vi "New Main Log Loop.vi"() -> ()   [LabVIEW 2015]
uses:
  packet types.ctl
  Main/Robot Global Data.vi
  <vilib>/Rock Robotics/WPI/Solenoid/Deprecated/WPI_SolenoidGetBool.vi
  <vilib>/Rock Robotics/WPI/Ultrasonic/WPI_SonarSRF04DigitalGetRange.vi
  <vilib>/Rock Robotics/WPI/Ultrasonic/WPI_UltrasonicRangeUnits.ctl
  <vilib>/Rock Robotics/WPI/CAN/Jaguar/SubVIs/WPI_CANJaguar_ControlMode.ctl
  <vilib>/Rock Robotics/WPI/CAN/TalonSRX/WPI_CANTalonSRX_APIControlMode.ctl
  <vilib>/Rock Robotics/SystemInterfaces/DIO/FPGA_DIOPWMChannel.ctl
  <vilib>/Rock Robotics/WPI/PWM/WPI_PWMDeadband.ctl
  <vilib>/Rock Robotics/WPI/MotorControl/WPI_MotorControlType.ctl
  <vilib>/Rock Robotics/WPI/MotorControl/WPI_MotorControlDeviceRef.ctl
  <vilib>/Rock Robotics/WPI/Solenoid/WPI_SolenoidChannel.ctl
  <vilib>/Rock Robotics/WPI/Solenoid/WPI_SolenoidDevRef.ctl
  <vilib>/Rock Robotics/SystemInterfaces/DIO/FPGA_DIOChannel.ctl
  <vilib>/Rock Robotics/SystemInterfaces/Counter/FPGA_CounterCtrSystemIndex.ctl
  <vilib>/Rock Robotics/WPI/Ultrasonic/WPI_UltrasonicDeviceRef.ctl
  <vilib>/Rock Robotics/WPI/Compressor/WPI_CompressorDevRef.ctl
panel:
  in  "UltrasonicDevRef 2":T1={"DevStatus"={"status"=FALSE, "code"=0, "source"=""}, "Ping Channel"=enum."Invalid", "Echo Channel"=enum."Invalid", "CntIndex"=enum."Invalid"}
  in  "CompressorDevRef":T4
  in  "UltrasonicDevRef":T1={"DevStatus"={"status"=FALSE, "code"=0, "source"=""}, "Ping Channel"=enum."Invalid", "Echo Channel"=enum."Invalid", "CntIndex"=enum."Invalid"}
  out "error out":errorcluster
  out "result string":string
  in  "Piston 2 & 3 Val":T5={"DevStatus"={"status"=FALSE, "code"=0, "source"=""}, "Pneumatics Control Module"=0, "Forward Solenoid Channel"=enum."Invalid", "Reverse Solenoid Channel"=enum."Invalid"}
  in  "Piston 1 Val":T5={"DevStatus"={"status"=FALSE, "code"=0, "source"=""}, "Pneumatics Control Module"=0, "Forward Solenoid Channel"=enum."Invalid", "Reverse Solenoid Channel"=enum."Invalid"}
  in  "Collector Motor":T7={"DeviceStatus"={"status"=FALSE, "code"=0, "source"=""}, "Type"=enum."PWM", "PWM"={"PWM Channel"=enum."Invalid", "DeadBand"={"Name"="", "maxPositivePwm"=0, "minPositivePwm"=0, "centerPwm"=0, "maxNegativePwm"=0, "minNegativePwm"=0, "angularRange"=0}}, "CAN"={"Device Number"=0, "Control Mode"=enum."Percent VBus", "Semaphore"=refnum, "Max Vout"=12.0, "TalonSRX Control Mode"=enum."Percent VBus"}, "Invert"=FALSE}
  in  "Left Drive Motor":T7={"DeviceStatus"={"status"=FALSE, "code"=0, "source"=""}, "Type"=enum."PWM", "PWM"={"PWM Channel"=enum."Invalid", "DeadBand"={"Name"="", "maxPositivePwm"=0, "minPositivePwm"=0, "centerPwm"=0, "maxNegativePwm"=0, "minNegativePwm"=0, "angularRange"=0}}, "CAN"={"Device Number"=0, "Control Mode"=enum."Percent VBus", "Semaphore"=refnum, "Max Vout"=12.0, "TalonSRX Control Mode"=enum."Percent VBus"}, "Invert"=FALSE}
  in  "Right Drive Motor":T7={"DeviceStatus"={"status"=FALSE, "code"=0, "source"=""}, "Type"=enum."PWM", "PWM"={"PWM Channel"=enum."Invalid", "DeadBand"={"Name"="", "maxPositivePwm"=0, "minPositivePwm"=0, "centerPwm"=0, "maxNegativePwm"=0, "minNegativePwm"=0, "angularRange"=0}}, "CAN"={"Device Number"=0, "Control Mode"=enum."Percent VBus", "Semaphore"=refnum, "Max Vout"=12.0, "TalonSRX Control Mode"=enum."Percent VBus"}, "Invert"=FALSE}
  in  "Right CAN Drive Motor":T7={"DeviceStatus"={"status"=FALSE, "code"=0, "source"=""}, "Type"=enum."PWM", "PWM"={"PWM Channel"=enum."PWM 1", "DeadBand"={"Name"="", "maxPositivePwm"=0, "minPositivePwm"=0, "centerPwm"=0, "maxNegativePwm"=0, "minNegativePwm"=0, "angularRange"=0}}, "CAN"={"Device Number"=0, "Control Mode"=enum."Percent VBus", "Semaphore"=refnum, "Max Vout"=12.0, "TalonSRX Control Mode"=enum."Percent VBus"}, "Invert"=FALSE}
  in  "Collector CAN Motor":T7={"DeviceStatus"={"status"=FALSE, "code"=0, "source"=""}, "Type"=enum."PWM", "PWM"={"PWM Channel"=enum."PWM 1", "DeadBand"={"Name"="", "maxPositivePwm"=0, "minPositivePwm"=0, "centerPwm"=0, "maxNegativePwm"=0, "minNegativePwm"=0, "angularRange"=0}}, "CAN"={"Device Number"=0, "Control Mode"=enum."Percent VBus", "Semaphore"=refnum, "Max Vout"=12.0, "TalonSRX Control Mode"=enum."Percent VBus"}, "Invert"=FALSE}
  in  "Left CAN Drive Motor":T7={"DeviceStatus"={"status"=FALSE, "code"=0, "source"=""}, "Type"=enum."PWM", "PWM"={"PWM Channel"=enum."PWM 1", "DeadBand"={"Name"="", "maxPositivePwm"=0, "minPositivePwm"=0, "centerPwm"=0, "maxNegativePwm"=0, "minNegativePwm"=0, "angularRange"=0}}, "CAN"={"Device Number"=0, "Control Mode"=enum."Percent VBus", "Semaphore"=refnum, "Max Vout"=12.0, "TalonSRX Control Mode"=enum."Percent VBus"}, "Invert"=FALSE}
  in  "error in (no error)":errorcluster
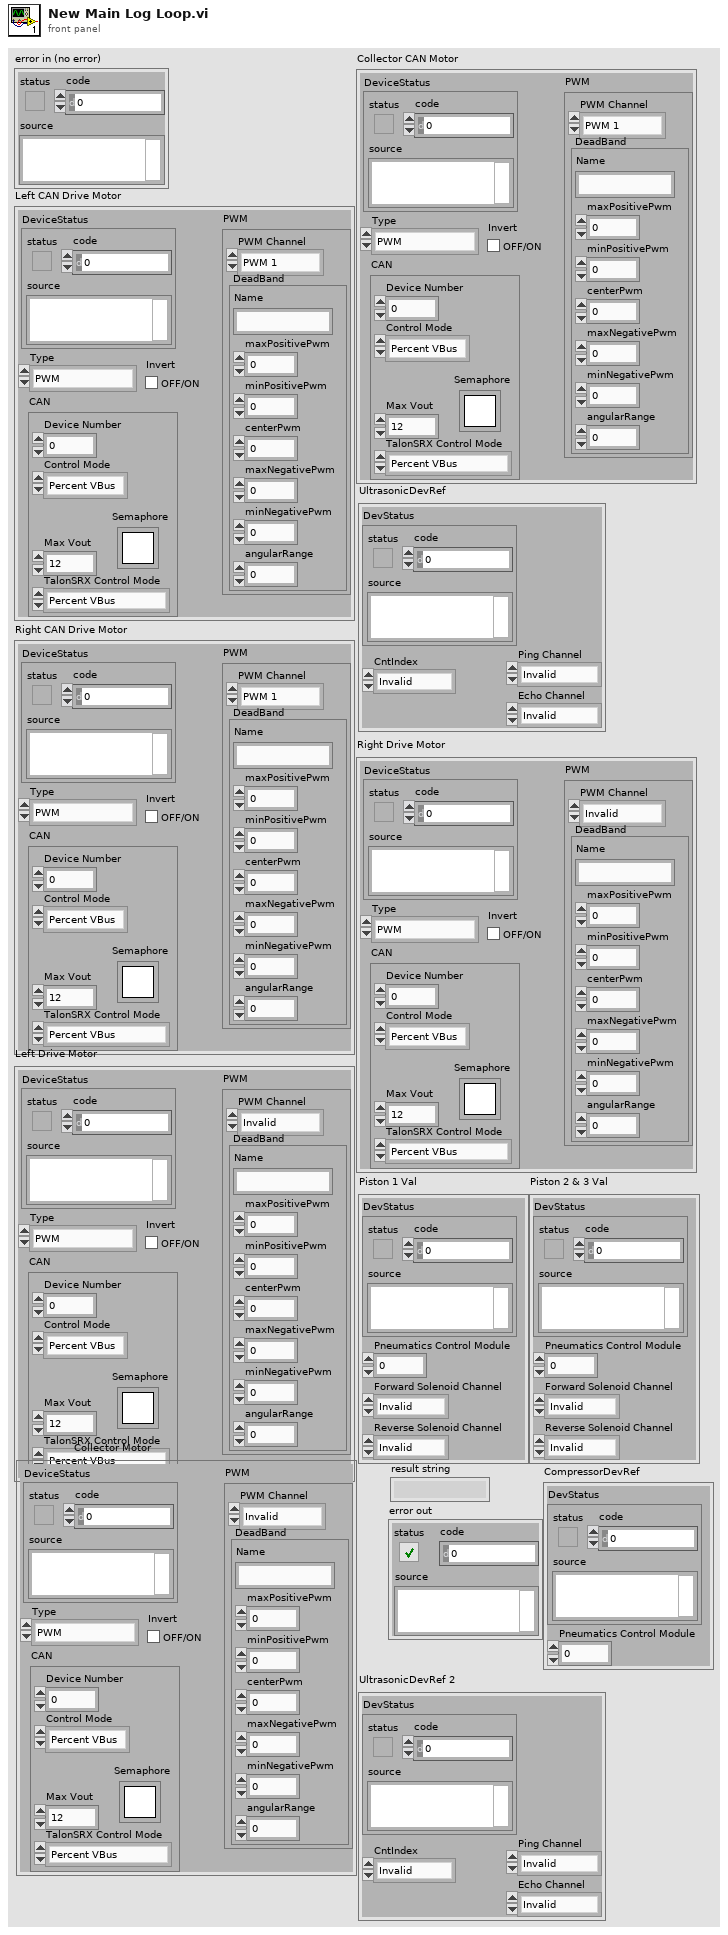
[diagram p1: front panel]
types:
  T1 = typedef "WPI_UltrasonicDeviceRef.ctl" = cluster{"DevStatus":errorcluster, "Ping Channel":T2, "Echo Channel":T2, "CntIndex":T3}
  T2 = typedef "FPGA_DIOChannel.ctl" = enum8{"DIO 0", "DIO 1", "DIO 2", "DIO 3", "DIO 4", "DIO 5", "DIO 6", "DIO 7", "DIO 8", "DIO 9", "DIO MXP 0", "DIO MXP 1", "DIO MXP 2", "DIO MXP 3", "DIO MXP 4", "DIO MXP 5", "DIO MXP 6", "DIO MXP 7", "DIO MXP 8", "DIO MXP 9", "DIO MXP 10", "DIO MXP 11", "DIO MXP 12", "DIO MXP 13", "DIO MXP 14", "DIO MXP 15", "Invalid"}
  T3 = typedef "FPGA_CounterCtrSystemIndex.ctl" = enum8{"Ctr 0", "Ctr 1", "Ctr 2", "Ctr 3", "Ctr 4", "Ctr 5", "Ctr 6", "Ctr 7", "Invalid"}
  T4 = typedef "WPI_CompressorDevRef.ctl" = cluster{"DevStatus":errorcluster, "Pneumatics Control Module":u8}
  T5 = typedef "WPI_SolenoidDevRef.ctl" = cluster{"DevStatus":errorcluster, "Pneumatics Control Module":u8, "Forward Solenoid Channel":T6, "Reverse Solenoid Channel":T6}
  T6 = typedef "WPI_SolenoidChannel.ctl" = enum8{"Solenoid 0", "Solenoid 1", "Solenoid 2", "Solenoid 3", "Solenoid 4", "Solenoid 5", "Solenoid 6", "Solenoid 7", "Invalid"}
  T7 = typedef "WPI_MotorControlDeviceRef.ctl" = cluster{"DeviceStatus":errorcluster, "Type":T8, "PWM":cluster{"PWM Channel":T9, "DeadBand":T10}, "CAN":cluster{"Device Number":u8, "Control Mode":T11, "Semaphore":T12, "Max Vout":dbl, "TalonSRX Control Mode":T13}, "Invert":bool}
  T8 = typedef "WPI_MotorControlType.ctl" = enum16{"PWM", "CAN", "CANTalonSRX"}
  T9 = typedef "FPGA_DIOPWMChannel.ctl" = enum8{"PWM 0", "PWM 1", "PWM 2", "PWM 3", "PWM 4", "PWM 5", "PWM 6", "PWM 7", "PWM 8", "PWM 9", "PWM MXP 0", "PWM MXP 1", "PWM MXP 2", "PWM MXP 3", "PWM MXP 4", "PWM MXP 5", "PWM MXP 6", "PWM MXP 7", "PWM MXP 8", "PWM MXP 9", "Invalid"}
  T10 = typedef "WPI_PWMDeadband.ctl" = cluster{"Name":string, "maxPositivePwm":i32, "minPositivePwm":i32, "centerPwm":i32, "maxNegativePwm":i32, "minNegativePwm":i32, "angularRange":u16}
  T11 = typedef "WPI_CANJaguar_ControlMode.ctl" = enum8{"Percent VBus", "Current", "Speed", "Position", "Voltage"}
  T12 = typedef "Semaphore RefNum" = refnum<k1>
  T13 = typedef "WPI_CANTalonSRX_APIControlMode.ctl" = enum8{"Percent VBus", "Speed", "Position", "Slave", "Unchanged / Invalid", "Voltage Compensation", "Current", "Motion Profile"}
  T14 = typedef "packet types.ctl" = enum16{"Log line", "Open File", "Send Header", "Set Time", "Send to LCD"}
  T15 = typedef "WPI_SerialPortRef.ctl" = cluster{"DevStatus":errorcluster, "Serial Port Name":refnum<visa-resource-name>}
  T16 = typedef "WPI_UltrasonicRangeUnits.ctl" = enum16{"inches", "mm"}
  T17 = typedef "WPI_DriverStationRobotMode2.ctl" = enum16{"Autonomous Disabled", "Autonomous Enabled", "Teleop Disabled", "Teleop Enabled", "Disconnected", "Finish", "Test Disabled", "Test Enabled", "Emergency Stopped"}
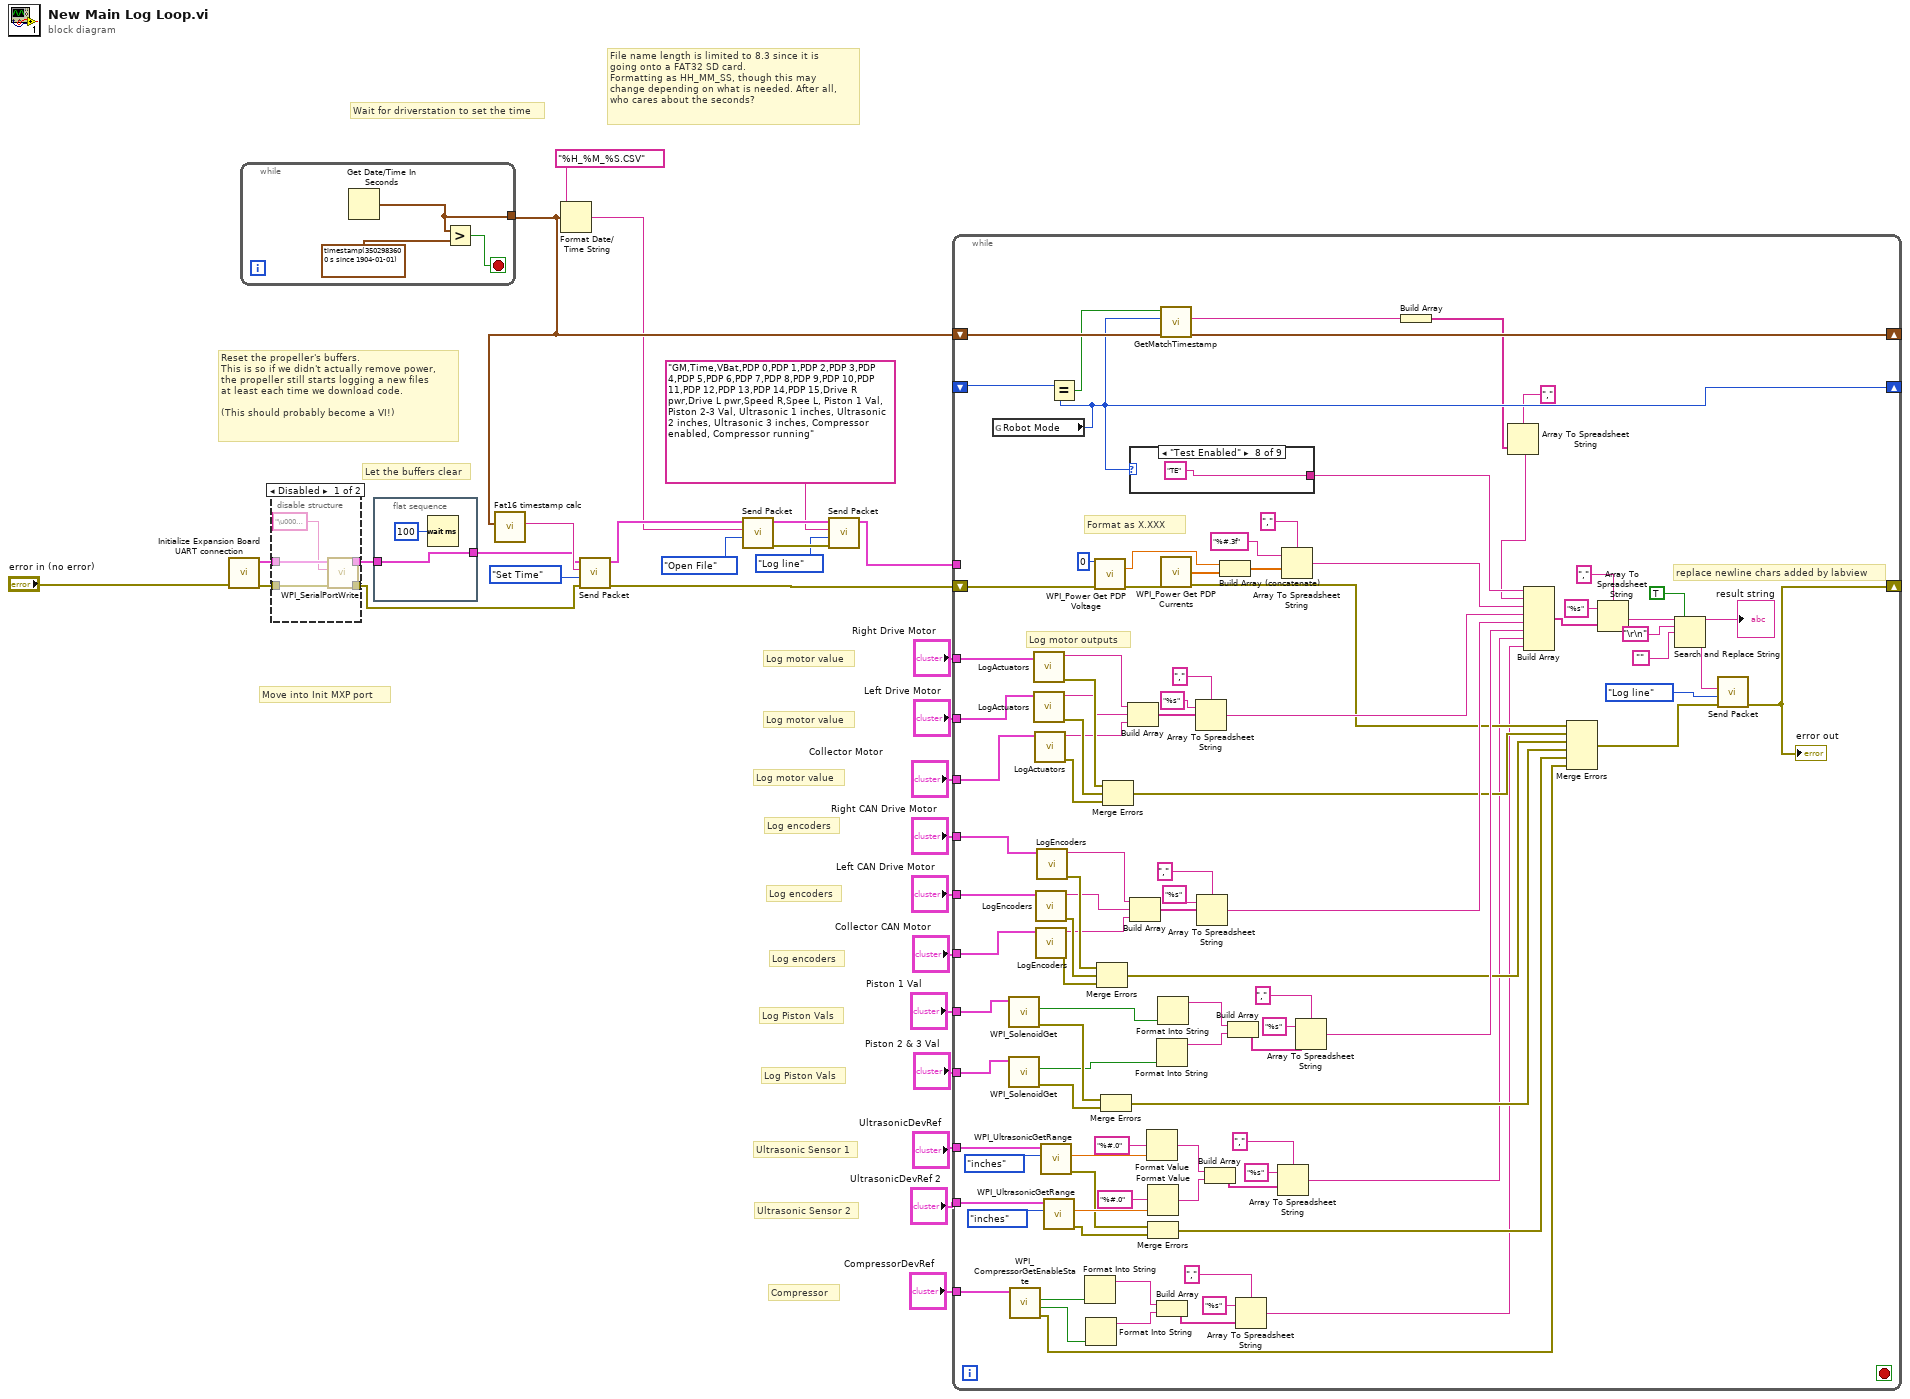
[diagram p0: block diagram]
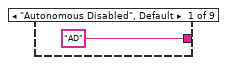
[diagram p2: hidden frame]
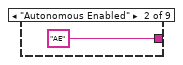
[diagram p3: hidden frame]
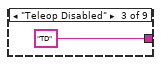
[diagram p4: hidden frame]
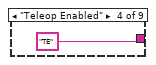
[diagram p5: hidden frame]
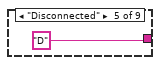
[diagram p6: hidden frame]
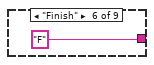
[diagram p7: hidden frame]
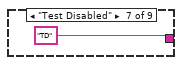
[diagram p8: hidden frame]
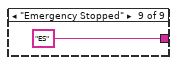
[diagram p9: hidden frame]
diagram:
  # "Compressor"
  # "Ultrasonic Sensor 2"
  # "Ultrasonic Sensor 1"
  # "Log motor value"
  # "Log motor value"
  # "Log motor value"
  # "Log encoders"
  # "Log encoders"
  # "Log Piston Vals"
  # "Log Piston Vals"
  # "Log encoders"
  # "Move into Init MXP port"
  # "Let the buffers clear"
  # "Reset the propeller's buffers.\nThis is so if we didn't actually remove power,\nthe propeller still starts logging a new files \nat least each time we download code.\n\n(This should probably become a VI!)"
  # "File name length is limited to 8.3 since it is \ngoing onto a FAT32 SD card. \nFormatting as HH_MM_SS, though this may\nchange depending on what is needed. After all,\nwho cares about the seconds?"
  # "Wait for driverstation to set the time"
  n1 = call "Initialize Expansion Board UART connection.vi"("error in (no error)"="error in (no error)") -> ("error out"=w27:errorcluster, "SerialPortRef"=w26:T15)  [unwired: 9 in]
  n2 = while {
    tunnel: [w31] -> w18
    stop <- w32 stop-if-true
    n3 = Get Date/Time In Seconds() -> (seconds since 1Jan1904=w31:timestamp)
    n4 = Greater?(x=w31, y=timestamp(3502983600 s since 1904-01-01)) -> (0:w32:bool)
  }
  n5 = disable-structure shown="Disabled" {
    disable-tunnel: w27 -> [w38 w39]
    disable-tunnel: w26 -> [w37 w40]
    disable-tunnel: [w35 w40] -> w24
    disable-tunnel: [w34 w39] -> w23
    frame Disabled {
      n6 = call <vilib>:"WPI_SerialPortWrite.vi"("error in (no error)"=w38, "Buffer"="\u0004\u0004", "SerialPortRef"=w37) -> ("error out"=w34:errorcluster, "SerialPortRef"=w35:T15)  [unwired: 6 in, 1 out]
    }
    frame Enabled {
    }
  }
  n7 = flat-sequence {
    tunnel: [w42] -> w25
    tunnel: w24 -> [w42]
    frame #0 {
      n8 = Wait (ms)(milliseconds to wait=u32 100) -> ()  [unwired: 1 out]
    }
  }
  n9 = call "Fat16 timestamp calc.vi"("time stamp"=w18) -> ("timestamp as string"=w29:string)  [unwired: 10 in]
  n10 = Format Date/Time String(time format string (%c)="%H_%M_%S.CSV", seconds (now)=w18) -> (date/time string=w11:string)  [unwired: 1 in]
  n11 = call "Send Packet.vi"("error in (no error)"=w23, 7:packet_types."Set Time", "Log string"=w29, "SerialPortRef"=w25) -> ("error out"=w4:errorcluster, "SerialPortRef out"=w12:T15)  [unwired: 4 in]
  n12 = call "Send Packet.vi"(7:packet_types."Open File", "Log string"=w11, "SerialPortRef"=w12) -> ("error out"=w16:errorcluster, "SerialPortRef out"=w17:T15)  [unwired: 5 in]
  n13 = call "Send Packet.vi"("error in (no error)"=w16, 7:packet_types."Log line", "Log string"="GM,Time,VBat,PDP 0,PDP 1,PDP 2,PDP 3,PDP 4,PDP 5,PDP 6,PDP 7,PDP 8,PDP 9,PDP 10,PDP 11,PDP 12,PDP 13,PDP 14,PDP 15,Drive R pwr,Drive L pwr,Speed R,Spee L, Piston 1 Val, Piston 2-3 Val, Ultrasonic 1 inches, Ultrasonic 2 inches, Ultrasonic 3 inches, Compressor enabled, Compressor running", "SerialPortRef"=w17) -> ("SerialPortRef out"=w13:T15)  [unwired: 4 in, 1 out]
  n14 = while {
    tunnel: "Left CAN Drive Motor" -> [w141]
    tunnel: "Collector CAN Motor" -> [w140]
    tunnel: "Right CAN Drive Motor" -> [w139]
    shift-right: [w135] -> _
    shift-left: w18 -> [w134]
    shift-right: [w131] -> _
    shift-left: _ -> [w133]
    tunnel: w13 -> [_]
    tunnel: "Right Drive Motor" -> [w114]
    tunnel: "Left Drive Motor" -> [w113]
    tunnel: "Collector Motor" -> [w112]
    tunnel: "Piston 1 Val" -> [w101]
    tunnel: "Piston 2 & 3 Val" -> [w100]
    shift-right: [w77] -> _
    shift-left: w4 -> [w76]
    tunnel: "UltrasonicDevRef" -> [w75]
    tunnel: "CompressorDevRef" -> [w71]
    tunnel: "UltrasonicDevRef 2" -> [w68]
    stop <- _ stop-if-true
    # "replace newline chars added by labview"
    # "Log motor outputs"
    # "Format as X.XXX"
    n15 = global read "Robot Global Data.vi" "Robot Mode"() -> (w131:T17)
    n16 = call-poly <vilib>:"WPI_SolenoidGet.vi"("SolenoidDevRef"=w101) -> ("error out"=w98:errorcluster, "Value"=w97:bool)  [unwired: 8 in, 1 out]
    n17 = call-poly <vilib>:"WPI_SolenoidGet.vi"("SolenoidDevRef"=w100) -> ("error out"=w99:errorcluster, "Value"=w96:bool)  [unwired: 8 in, 1 out]
    n18 = call <vilib>:"WPI_CompressorGetEnableState.vi"("CompressorDevRef"=w71) -> ("error out"=w51:errorcluster, "Compressor Running"=w53:bool, "Enabled"=w54:bool)  [unwired: 7 in, 1 out]
    n19 = call "LogActuators.vi"("MotorControlDevRef"=w114) -> ("error out"=w109:errorcluster, "resulting string"=w106:string)  [unwired: 9 in]
    n20 = call "LogActuators.vi"("MotorControlDevRef"=w113) -> ("error out"=w110:errorcluster, "resulting string"=w105:string)  [unwired: 9 in]
    n21 = call "LogActuators.vi"("MotorControlDevRef"=w112) -> ("error out"=w111:errorcluster, "resulting string"=w104:string)  [unwired: 9 in]
    n22 = call "LogEncoders.vi"("CAN Talon SRX Ref"=w141) -> ("error out"=w137:errorcluster, "concatenated string"=w126:string)  [unwired: 9 in]
    n23 = call "LogEncoders.vi"("CAN Talon SRX Ref"=w140) -> ("error out"=w136:errorcluster, "concatenated string"=w125:string)  [unwired: 9 in]
    n24 = call "LogEncoders.vi"("CAN Talon SRX Ref"=w139) -> ("error out"=w138:errorcluster, "concatenated string"=w127:string)  [unwired: 9 in]
    n25 = call-poly <vilib>:"WPI_UltrasonicGetRange.vi"("Range Units"=WPI_UltrasonicRangeUnits."inches", "UltrasonicDevRef"=w75) -> ("error out"=w61:errorcluster, "Distance"=w72:dbl)  [unwired: 7 in, 1 out]
    n26 = call-poly <vilib>:"WPI_UltrasonicGetRange.vi"("Range Units"=WPI_UltrasonicRangeUnits."inches", "UltrasonicDevRef"=w68) -> ("error out"=w60:errorcluster, "Distance"=w69:dbl)  [unwired: 7 in, 1 out]
    n27 = Equal?(x=w133, y=w131) -> (x = y?=w132:bool)
    n28 = Format Into String(w54) -> (resulting string=w57:string)  [unwired: 3 in, 1 out]
    n29 = Format Into String(w53) -> (resulting string=w56:string)  [unwired: 3 in, 1 out]
    n30 = call <vilib>:"WPI_Power Get PDP Voltage.vi"("Power Distribution Panel (0)"=u8 0, "error in"=w76) -> ("voltage (V)"=w121:dbl, "error out"=w118:errorcluster)  [unwired: 12 in]
    n31 = Merge Errors(w138, w137, w136) -> (w80:errorcluster)
    n32 = Merge Errors(w98, w99) -> (w79:errorcluster)
    n33 = Merge Errors(w109, w110, w111) -> (w81:errorcluster)
    n34 = Build Array(w106, w105, w104) -> (w108:string[])
    n35 = case shown="\"Test Enabled\"" w131 {
      tunnel: ["AD" "AE" "TD" "TE" "D" "F" "TD" "TE" "ES"] -> w130
      frame "Autonomous Disabled", Default {
      }
      frame "Autonomous Enabled" {
      }
      frame "Teleop Disabled" {
      }
      frame "Teleop Enabled" {
      }
      frame "Disconnected" {
      }
      frame "Finish" {
      }
      frame "Test Disabled" {
      }
      frame "Test Enabled" {
      }
      frame "Emergency Stopped" {
      }
    }
    n36 = Build Array(w127, w126, w125) -> (w129:string[])
    n37 = Format Value(format string="%#.0", value (0)=w72) -> (output string=w64:string)  [unwired: 1 in]
    n38 = Format Value(format string="%#.0", value (0)=w69) -> (output string=w63:string)  [unwired: 1 in]
    n39 = Merge Errors(w61, w60) -> (w59:errorcluster)
    n40 = Format Into String(w96) -> (resulting string=w93:string)  [unwired: 3 in, 1 out]
    n41 = Build Array(w57, w56) -> (w58:string[])
    n42 = Format Into String(w97) -> (resulting string=w94:string)  [unwired: 3 in, 1 out]
    n43 = call "GetMatchTimestamp.vi"("seconds since 1Jan1904"=w134, "Robot Mode"=w131, "Boolean"=w132) -> ("seconds since 1Jan1904 2"=w135:timestamp, "Match Timestamp"=w44:string)  [unwired: 7 in]
    n44 = call <vilib>:"WPI_Power Get PDP Currents.vi"("error in"=w118) -> ("all currents (A)"=w119:dbl[], "error out"=w82:errorcluster)  [unwired: 12 in, 1 out]
    n45 = Array To Spreadsheet String(delimiter (Tab)=",", array=w108, 3:"%s" ("format string")) -> (spreadsheet string=w102:string)
    n46 = Array To Spreadsheet String(delimiter (Tab)=",", array=w129, 3:"%s" ("format string")) -> (spreadsheet string=w103:string)
    n47 = Build Array(w64, w63) -> (w66:string[])
    n48 = Build Array (concatenate)(w121, w119) -> (w120:dbl[])
    n49 = Build Array(w94, w93) -> (w95:string[])
    n50 = Array To Spreadsheet String(delimiter (Tab)=",", array=w58, 3:"%s" ("format string")) -> (spreadsheet string=w52:string)
    n51 = Array To Spreadsheet String(delimiter (Tab)=",", array=w66, 3:"%s" ("format string")) -> (spreadsheet string=w62:string)
    n52 = Array To Spreadsheet String(delimiter (Tab)=",", array=w120, 3:"%#.3f" ("format string")) -> (spreadsheet string=w117:string)
    n53 = Array To Spreadsheet String(delimiter (Tab)=",", array=w95, 3:"%s" ("format string")) -> (spreadsheet string=w91:string)
    n54 = Build Array(w44) -> (w43:string[])
    n55 = Array To Spreadsheet String(delimiter (Tab)=",", array=w43) -> (spreadsheet string=w116:string)  [unwired: 1 in]
    n56 = Build Array(w130, w116, w117, w102, w103, w91, w62, w52) -> (w85:string[])
    n57 = Merge Errors(w82, w81, w80, w79, w59, w51) -> (w78:errorcluster)
    n58 = Array To Spreadsheet String(delimiter (Tab)=",", array=w85, 3:"%s" ("format string")) -> (spreadsheet string=w86:string)
    n59 = Search and Replace String(replace all?=TRUE ("replace all? (F)"), input string=w86, search string="\r\n", replace string="") -> (result string=w84:string)  [unwired: 4 in, 3 out]
    "result string" <- w84
    n60 = call "Send Packet.vi"("error in (no error)"=w78, 7:packet_types."Log line", "Log string"=w84) -> ("error out"=w77:errorcluster)  [unwired: 5 in, 1 out]
    "error out" <- w77
  }
